vi "rqcAlice QKey Processing.vi"(0 "rqcAlice ServiceNET in":T1, 1 "Sessions to Key File":u32, 5 "Bob's data":u32[](array[numeric]), 7 "Alice's Raw data":u8[](array[numeric]), 11 "error in (no error)":errorcluster, 12 "Write to File QBER threshold":dbl=5.0 format="%#_g %") -> (4 "rqcAlice ServiceNET out":T1, 6 "QBER, %":dbl[](array[numeric]), 13 "Bob's Key:":string="000001111000001000111001111011010101010110101010000001111011010111010100010111101101000100111011011011100011101010101111010000010101011111010011110111101011110110111011001100100110010000110101011100111010010011100011011100000100000100011001010111010011011011011111001000001100001100101000101111000011101010000011011101000010000001100110010111011010110010111010010100010111010010111010010010101000110110111000000101101000010001111111011110101110001110011010101111011010011001011111000111111101001100010111110011011101111001111000111010111111101001001100001111010010001111001011101101001000000101001010", 14 "Alice's Key:":string="000001111000001000111000111011010101010110101010000001111011010111010100010111101001000110111011011011100011101010101111010010010101011111010011110111101011111110111011001100100110010000110101011100111010010011100011011100000100000100011001110111010011011011011101001000001100001100101000101111000011100010000011011101000010000001100010110111011010110010111010010100010111010010111010010010101000110110111000000101101000010001111111011110101110001110011010101111011010011001011111000111111101001100010111110011011101111001111000111010111111101001001100001111010010001111001011111101001000000101001010", 15 "error out":errorcluster)   [LabVIEW 2018]
uses:
  Shared/Shared Host Lib/rqc ServiceNET/Alice/Custom Controls/rqcAlice ServiceNET control.ctl
  Custom Controls/rqcAlice QKey Processing Type.ctl
  Shared/Shared Host Lib/rqc ServiceNET/Custom Controls/rqc ServiceNET command.ctl
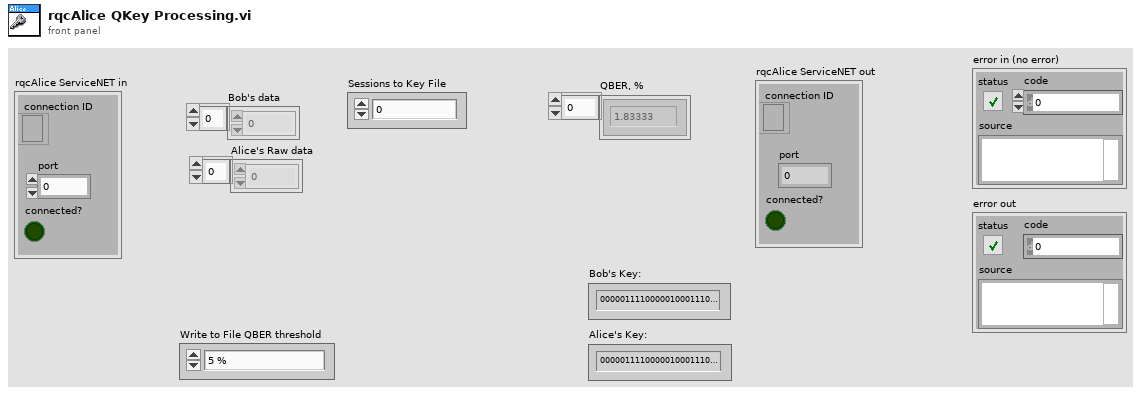
[diagram p1: front panel]
types:
  T1 = typedef "rqcAlice ServiceNET control.ctl" = cluster{"connection ID":refnum<k5>, "port":u16, "connected?":bool}
  T2 = typedef "rqcAlice QKey Processing Type.ctl" = enum16{"usual", "Key File"}
  T3 = typedef "rqc ServiceNET command.ctl" = enum8{"NONE", "READY", "START", "PING", "SEND KEY", "WRITE KEY", "WRITE AND SAVE KEY"}
  T4 = enum16{"open", "replace", "create", "open or create", "replace or create", "replace or create with confirmation"}
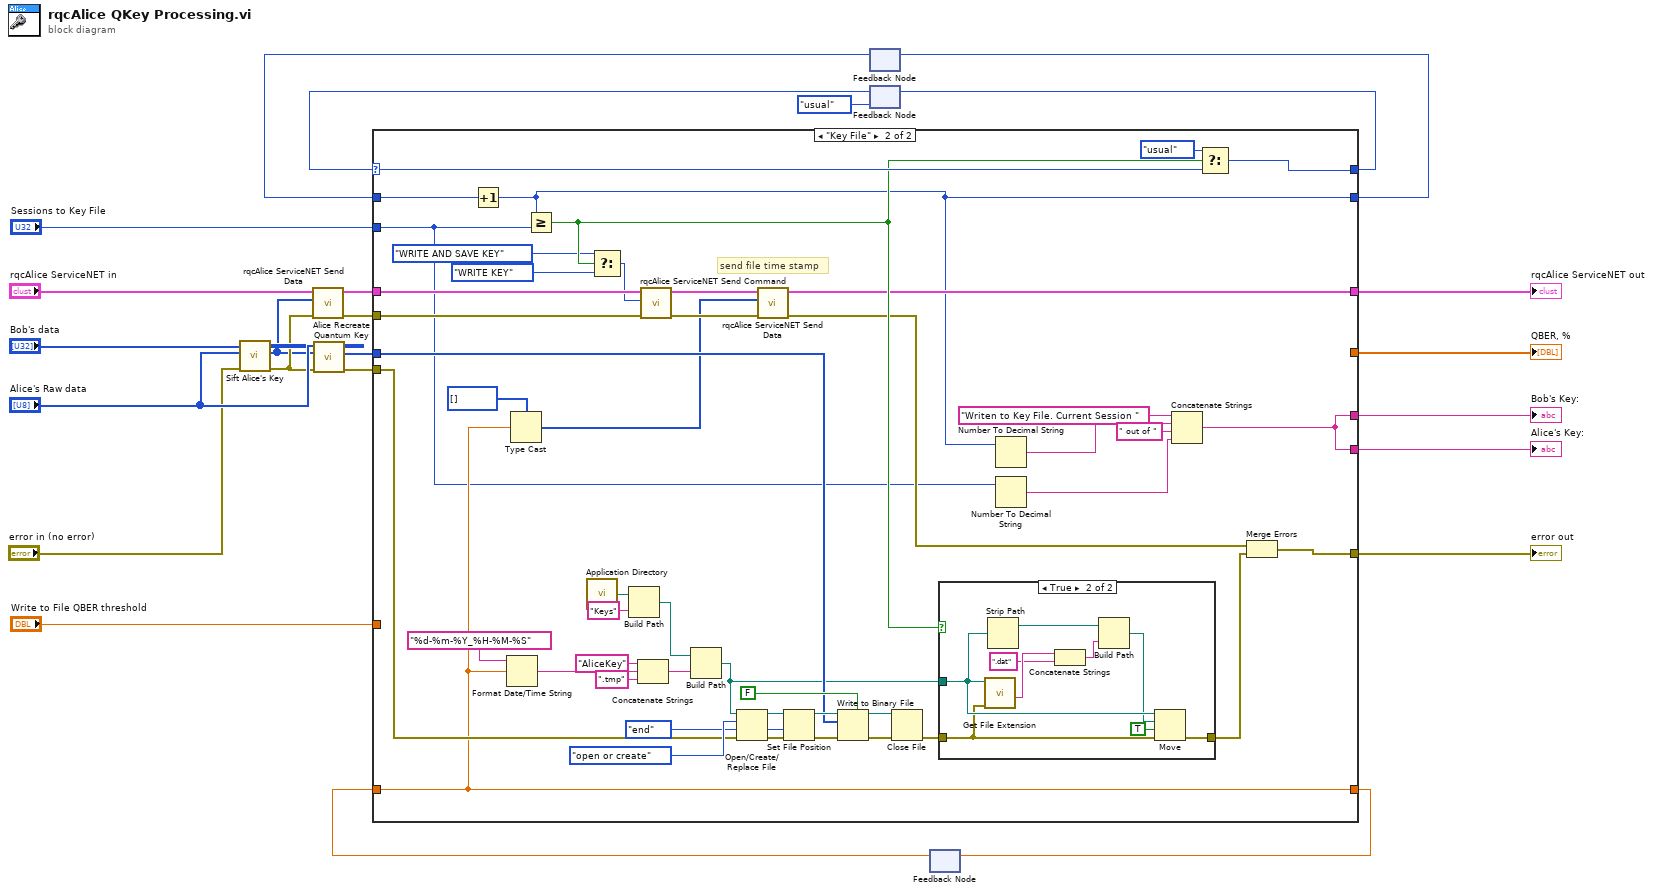
[diagram p0: block diagram]
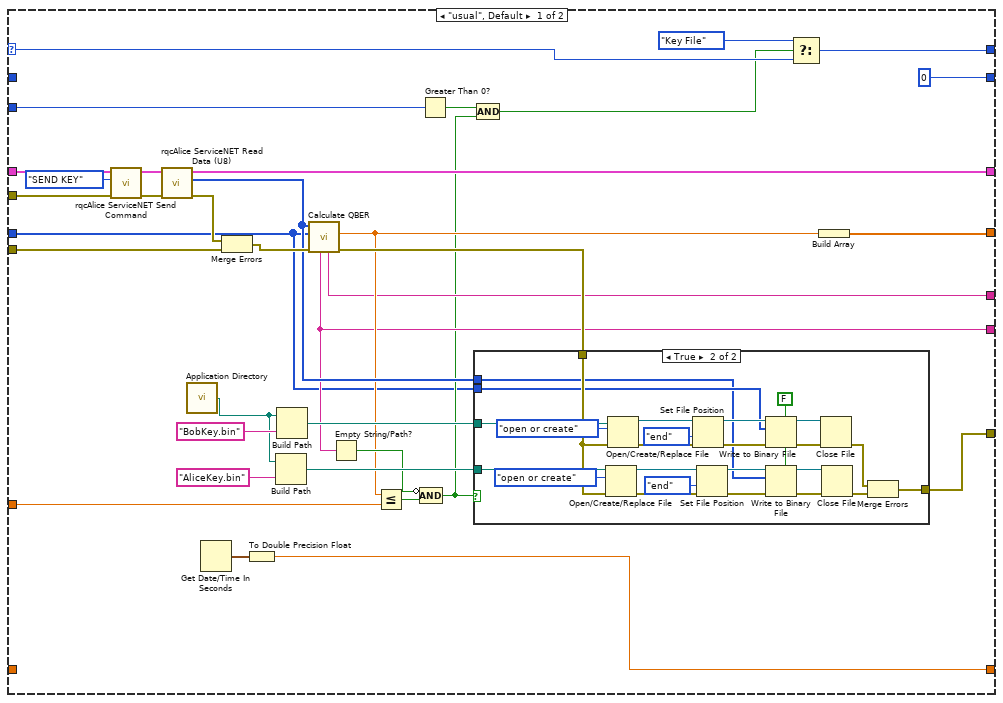
[diagram p2: hidden frame]
diagram:
  n1 = call "Sift Alice's Key.vi"("error in"="error in (no error)", "Alice's Raw Data in"="Alice's Raw data", "Bob's Data in"="Bob's data") -> ("error out"=w13:errorcluster, "Bob's correct measurements indexes"=w12:u32[])  [unwired: 6 in, 1 out]
  n2 = call "rqcAlice ServiceNET Send Data.vi"("error in"=w13, "Data"=w12, "rqcAlice ServiceNET in"="rqcAlice ServiceNET in") -> ("error out"=w9:errorcluster, "rqcAlice ServiceNET out"=w8:T1)  [unwired: 7 in]
  n3 = call "Alice Recreate Quantum Key.vi"("error in"=w13, "Correct Measurements Indexes in"=w12, "Raw Data in"="Alice's Raw data") -> ("error out"=w11:errorcluster, "Sifted Key out"=w10:u8[])  [unwired: 6 in, 1 out]
  n4 = feedback #1() -> (w1:u32)  [unwired: 1 in]
  n5 = feedback #2(rqcAlice_QKey_Processing_Type."usual" ("rqcAlice QKey Processing Type")) -> (w6:T2)
  n6 = feedback #3() -> (w3:dbl)  [unwired: 1 in]
  n7 = case shown="\"Key File\"" w6 {
    selector: w6 -> [w43 w122]
    tunnel: w8 -> [w31 w115]
    tunnel: [w59 w97] -> w20
    tunnel: [w51 w101] -> w23
    tunnel: [w25 _] -> w18
    tunnel: "Write to File QBER threshold" -> [w46 _]
    tunnel: [w45 w90] -> w16
    tunnel: [w44 w90] -> w15
    tunnel: [w42 w120] -> w5
    tunnel: "Sessions to Key File" -> [w40 w87]
    tunnel: w11 -> [w36 w106]
    tunnel: w10 -> [w35 w124]
    tunnel: w9 -> [w30 w114]
    tunnel: [w26 w94] -> w4
    tunnel: w3 -> [_ w94]
    tunnel: [u32 0 w91] -> w2
    tunnel: w1 -> [_ w123]
    frame "usual", Default {
      n8 = call "rqcAlice ServiceNET Send Command.vi"("error in"=w30, "command"=rqc_ServiceNET_command."SEND KEY", "rqcAlice ServiceNET in"=w31) -> ("error out"=w28:errorcluster, "rqcAlice ServiceNET out"=w29:T1)  [unwired: 7 in]
      n9 = call "rqcAlice ServiceNET Read Data (U8).vi"("error in"=w28, "rqcAlice ServiceNET in"=w29) -> ("error out"=w57:errorcluster, "data"=w48:u8[], "rqcAlice ServiceNET out"=w59:T1)  [unwired: 6 in, 1 out]
      n10 = call <vilib>:"Application Directory.vi"() -> ("Application Directory"=w34:path)
      n11 = Get Date/Time In Seconds() -> (seconds since 1Jan1904=w27:timestamp)
      n12 = Merge Errors(w57, w36) -> (w58:errorcluster)
      n13 = To Double Precision Float(number=w27) -> (double precision float=w26:dbl)
      n14 = Build Path(base path=w34, name or relative path="AliceKey.bin") -> (appended path=w53:path)
      n15 = Build Path(base path=w34, name or relative path="BobKey.bin") -> (appended path=w54:path)
      n16 = call "Calculate QBER.vi"("error in"=w58, "Alice's Key"=w35, "Bob's Key"=w48) -> ("error out"=w52:errorcluster, "QBER, %"=w47:dbl, "Bob's Key:"=w45:string, "Alice's Key:"=w44:string)  [unwired: 5 in]
      n17 = Empty String/Path?(string/path=w44) -> (empty?=w49:bool)
      n18 = Less Or Equal?(x=w47, y=w46) -> (x <= y?=w50:bool)
      n19 = Greater Than 0?(x=w40) -> (x > 0?=w39:bool)
      n20 = Compound Arithmetic op=AND(invert w49, w50) -> (w38:bool)
      n21 = case shown="True" w38 {
        tunnel: w54 -> [_ w85]
        tunnel: w53 -> [_ w82]
        tunnel: w52 -> [w60 w81]
        tunnel: [w60 w74] -> w51
        tunnel: w35 -> [_ w62]
        tunnel: w48 -> [_ w61]
        frame False {
        }
        frame True {
          w73 = FALSE ("prepend array or string size? (T)")
          n22 = Open/Create/Replace File(file path (use dialog)=w82, error in=w81, operation (0:open)=T4."open or create") -> (refnum out=w67:refnum<file>, error out=w63:errorcluster)  [unwired: 3 in, 1 out]
          n23 = Open/Create/Replace File(file path (use dialog)=w85, error in=w81, operation (0:open)=T4."open or create") -> (refnum out=w72:refnum<file>, error out=w70:errorcluster)  [unwired: 3 in, 1 out]
          n24 = Set File Position(refnum=w72, from (0:start)=enum16{"start", "end", "current"}."end", error in=w70) -> (refnum out=w71:refnum<file>, error out=w69:errorcluster)  [unwired: 1 in]
          n25 = Set File Position(refnum=w67, from (0:start)=enum16{"start", "end", "current"}."end", error in=w63) -> (refnum out=w66:refnum<file>, error out=w64:errorcluster)  [unwired: 1 in]
          n26 = Write to Binary File(file (use dialog)=w71, data=w62, error in=w69, 5:w73) -> (refnum out=w80:refnum<file>, error out=w79:errorcluster)  [unwired: 2 in, 1 out]
          n27 = Write to Binary File(file (use dialog)=w66, data=w61, error in=w64, 5:w73) -> (refnum out=w78:refnum<file>, error out=w77:errorcluster)  [unwired: 2 in, 1 out]
          n28 = Close File(refnum=w80, error in=w79) -> (error out=w76:errorcluster)  [unwired: 1 out]
          n29 = Close File(refnum=w78, error in=w77) -> (error out=w75:errorcluster)  [unwired: 1 out]
          n30 = Merge Errors(w76, w75) -> (w74:errorcluster)
        }
      }
      n31 = Compound Arithmetic op=AND(w39, w38) -> (w37:bool)
      n32 = Select(t=rqcAlice_QKey_Processing_Type."Key File", s=w37, f=w43) -> (s? t:f=w42:T2)
      n33 = Build Array(w47) -> (w25:dbl[])
    }
    frame "Key File" {
      # "send file time stamp"
      n34 = Increment(x=w123) -> (x+1=w91:u32)
      n35 = Format Date/Time String(time format string (%c)="%d-%m-%Y_%H-%M-%S", seconds (now)=w94) -> (date/time string=w99:string)  [unwired: 1 in]
      n36 = Type Cast(type=u32[] [], x=w94) -> (*(type *) &x=w92:u32[])
      n37 = Greater Or Equal?(x=w91, y=w87) -> (x >= y?=w104:bool)
      n38 = call <vilib>:"Application Directory.vi"() -> ("Application Directory"=w113:path)
      n39 = Select(t=rqc_ServiceNET_command."WRITE AND SAVE KEY", s=w104, f=rqc_ServiceNET_command."WRITE KEY" ("command")) -> (s? t:f=w103:T3)
      n40 = Build Path(base path=w113, name or relative path="Keys") -> (appended path=w110:path)
      n41 = Concatenate Strings("AliceKey" ("string"), w99, ".tmp" ("string")) -> (w109:string)
      n42 = call "rqcAlice ServiceNET Send Command.vi"("error in"=w114, "command"=w103, "rqcAlice ServiceNET in"=w115) -> ("error out"=w96:errorcluster, "rqcAlice ServiceNET out"=w98:T1)  [unwired: 7 in]
      n43 = Build Path(base path=w110, name or relative path=w109) -> (appended path=w111:path)
      n44 = Open/Create/Replace File(file path (use dialog)=w111, error in=w106, operation (0:open)=T4."open or create") -> (refnum out=w129:refnum<file>, error out=w127:errorcluster)  [unwired: 3 in, 1 out]
      n45 = call "rqcAlice ServiceNET Send Data.vi"("error in"=w96, "Data"=w92, "rqcAlice ServiceNET in"=w98) -> ("error out"=w95:errorcluster, "rqcAlice ServiceNET out"=w97:T1)  [unwired: 7 in]
      n46 = Set File Position(refnum=w129, from (0:start)=enum16{"start", "end", "current"}."end", error in=w127) -> (refnum out=w128:refnum<file>, error out=w126:errorcluster)  [unwired: 1 in]
      n47 = Write to Binary File(file (use dialog)=w128, data=w124, error in=w126, 5:FALSE ("prepend array or string size? (T)")) -> (refnum out=w119:refnum<file>, error out=w118:errorcluster)  [unwired: 2 in, 1 out]
      n48 = Close File(refnum=w119, error in=w118) -> (error out=w117:errorcluster)  [unwired: 1 out]
      n49 = case shown="True" w104 {
        tunnel: w111 -> [_ w141]
        tunnel: w117 -> [w133 w140]
        tunnel: [w133 w134] -> w116
        frame False {
        }
        frame True {
          n50 = call <vilib>:"Get File Extension.vi"("error in (no error)"=w140, "file"=w141) -> ("filename without extension"=w139:string)  [unwired: 5 in, 4 out]
          n51 = Strip Path(path=w141) -> (stripped path=w142:path)  [unwired: 1 out]
          n52 = Concatenate Strings(w139, ".dat" ("string")) -> (w137:string)
          n53 = Build Path(base path=w142, name or relative path=w137) -> (appended path=w136:path)
          n54 = Move(source path=w141, error in=w140, 9:TRUE ("overwrite (F)"), 10:w136) -> (error out=w134:errorcluster)  [unwired: 1 in, 2 out]
        }
      }
      n55 = Number To Decimal String(number=w91) -> (decimal integer string=w89:string)  [unwired: 1 in]
      n56 = Number To Decimal String(number=w87) -> (decimal integer string=w86:string)  [unwired: 1 in]
      n57 = Concatenate Strings("Writen to Key File. Current Session " ("Bob's Key:"), w89, " out of " ("string"), w86) -> (w90:string)
      n58 = Select(t=rqcAlice_QKey_Processing_Type."usual", s=w104, f=w122) -> (s? t:f=w120:T2)
      n59 = Merge Errors(w95, w116) -> (w101:errorcluster)
    }
  }
  "error out" <- w23
  "rqcAlice ServiceNET out" <- w20
  "QBER, %" <- w18
  "Bob's Key:" <- w16
  "Alice's Key:" <- w15
  n60 = feedback-in #1(w2) -> ()
  n61 = feedback-in #2(w5) -> ()
  n62 = feedback-in #3(w4) -> ()
